vi "testUintLessOrEqual.vi"(8 "error in (no error)":errorcluster, 11 "TestCase in":refnum<class "UnitTestUintClass.lvclass">) -> (0 "error out":errorcluster, 3 "TestCase out":refnum<class "UnitTestUintClass.lvclass">)   [LabVIEW 2011, in "UnitTestUintClass.lvclass"]
uses:
  UnitTestUintClass.lvclass
  UnitTestUintClass.lvclass/UnitTestUintClass.ctl
  <vilib>/addons/_JKI Toolkits/VI Tester/TestCase.llb/TestCase.lvclass
  UintClass/UintClass.lvclass
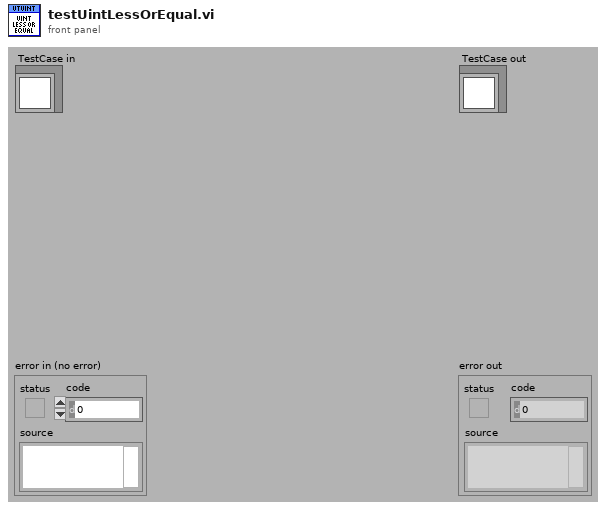
[diagram p1: front panel]
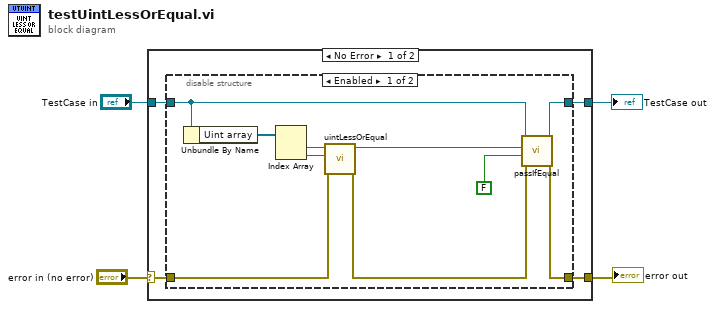
[diagram p0: block diagram]
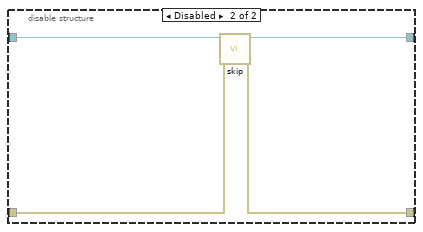
[diagram p2: hidden frame]
diagram:
  n1 = case shown="No Error" "error in (no error)" {
    selector: "error in (no error)" -> [w6 w24]
    tunnel: [w5 w24] -> w3
    tunnel: [w7 w23] -> w1
    tunnel: "TestCase in" -> [w8 w23]
    frame No Error {
      n2 = disable-structure shown="Enabled" {
        disable-tunnel: w8 -> [w16 w22]
        disable-tunnel: [w18 w19] -> w7
        disable-tunnel: w6 -> [w11 w21]
        disable-tunnel: [w17 w20] -> w5
        frame Enabled {
          n3 = Unbundle By Name(w16) -> ("Uint array"=w15:refnum<class "UintClass.lvclass">[])
          n4 = Index Array(array=w15) -> (element #1=w13:refnum<class "UintClass.lvclass">, element #2=w12:refnum<class "UintClass.lvclass">)  [unwired: 2 in]
          n5 = call "uintLessOrEqual.vi"("Error in (no error)"=w11, "Int2 in"=w12, "Int1 in"=w13) -> ("Error out"=w10:errorcluster, "Int1 <= Int2?"=w14:bool)  [unwired: 6 in, 1 out]
          n6 = call-dynamic "passIfEqual.vi"("error in (no error)"=w10, "y"=FALSE ("Int1 <= Int2?"), "x"=w14, "TestCase in"=w16) -> ("error out"=w17:errorcluster, "TestCase out"=w18:refnum<class "UnitTestUintClass.lvclass">)  [unwired: 6 in]
        }
        frame Disabled {
          n7 = call <vilib>:"skip.vi"("error in (no error)"=w21, "TestCase in"=w22) -> ("error out"=w20:errorcluster, "TestCase out"=w19:refnum<class "UnitTestUintClass.lvclass">)  [unwired: 8 in]
        }
      }
    }
    frame Error {
    }
  }
  "error out" <- w3
  "TestCase out" <- w1
